vi "HAL camera start acquire - SubVI.vi"(1 "error in":errorcluster) -> (0 "error out":errorcluster)   [LabVIEW 2014]
doc: "Starts an iXon acquisition (if not already running)"
uses:
  ATMCD32D.DLL
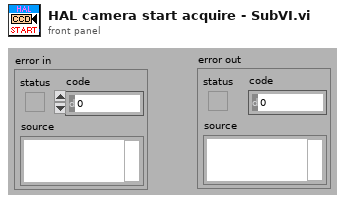
[diagram p1: front panel]
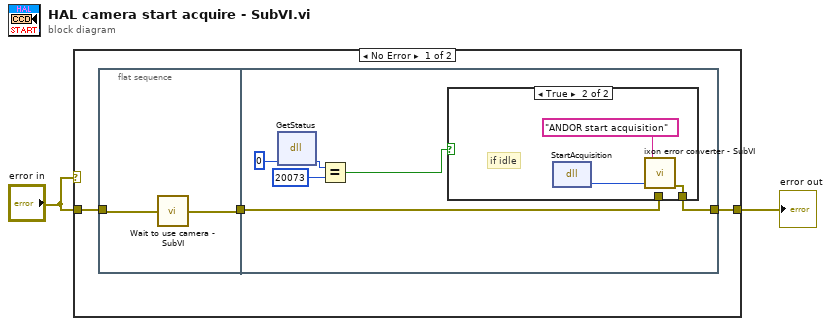
[diagram p0: block diagram]
diagram:
  n1 = case shown="No Error" "error in" {
    tunnel: "error in" -> [w5 w18]
    tunnel: [w4 w18] -> w2
    frame No Error {
      n2 = flat-sequence {
        tunnel: w5 -> [w6]
        tunnel: [w7] -> w3
        tunnel: [w8] -> w4
        tunnel: w3 -> [w13]
        frame #0 {
          n3 = call "Wait to use camera - SubVI.vi"("error in"=w6) -> ("error out"=w7:errorcluster)
        }
        frame #1 {
          n4 = dll-call lib="Atmcd32d.dll" fn="GetStatus" label="Call Library Function GetStatus"(u16 0) -> (w10:u32)  [unwired: 3 in, 3 out]
          n5 = Equal?(x=w10, y=u32 20073) -> (x = y?=w12:bool)
          n6 = case shown="True" w12 {
            tunnel: [w14 w15] -> w8
            tunnel: w13 -> [w14 _]
            frame False {
            }
            frame True {
              # "if idle"
              n7 = dll-call lib="Atmcd32d.dll" fn="StartAcquisition" label="start acquisition"() -> (w16:u32)  [unwired: 3 in, 2 out]
              n8 = call "ixon error converter - SubVI.vi"("Andor error code"=w16, "source"="ANDOR start acquisition") -> ("error out"=w15:errorcluster)  [unwired: 5 in]
            }
          }
        }
      }
    }
    frame Error {
    }
  }
  "error out" <- w2
